vi "Remove XLSX last empty row.vi"(8 "Error In":errorcluster, 11 "Array in":string[][](array[string])) -> (0 "Error Out":errorcluster, 1 "Last Empty Row Removed":bool, 3 "Array out":string[][](array[string]))   [LabVIEW 2021, in "Files.lvlib"]
uses:
  <userlib>/_OpenG.lib/array/array.llb/Remove Duplicates from 1D Array (String)__ogtk.vi
  Files.lvlib
  <userlib>/_OpenG.lib/array/array.llb/openg_array.lvlib
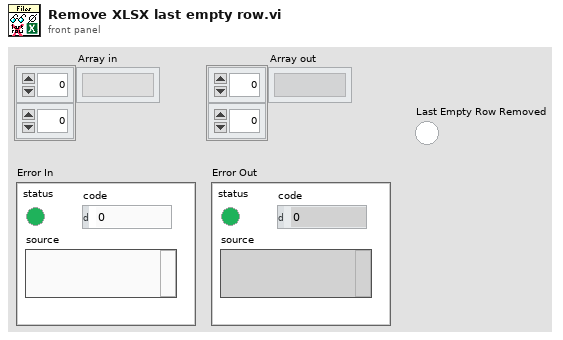
[diagram p1: front panel]
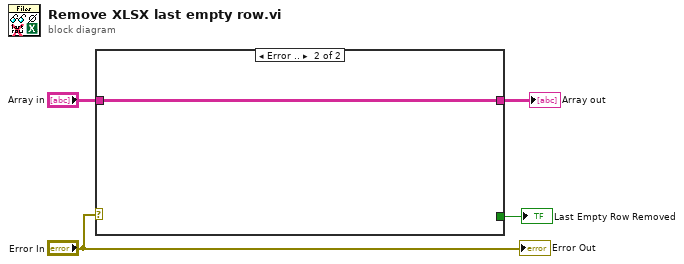
[diagram p0: block diagram]
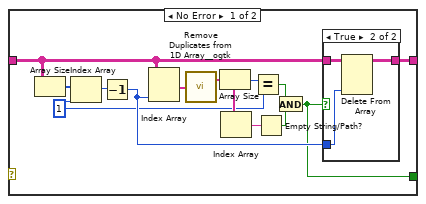
[diagram p2: hidden frame]
diagram:
  n1 = case shown="Error .." "Error In" {
    tunnel: "Array in" -> [w9 w22]
    tunnel: [w6 w22] -> w3
    tunnel: [w5 _] -> w2
    frame No Error {
      w12 = 1 ("index")
      n2 = Array Size(array=w9) -> (size(s)=w7:i32[])
      n3 = Index Array(array=w7, index=w12) -> (element=w8:i32)
      n4 = Decrement(x=w8) -> (x-1=w17:i32)
      n5 = Index Array(array=w9, index (col)=w17) -> (element=w10:string[])  [unwired: 1 in]
      n6 = call-poly <userlib>:"Remove Duplicates from 1D Array__ogtk.vi"("Input Array"=w10) -> ("Output Array"=w13:string[])  [unwired: 1 out]
      n7 = Array Size(array=w13) -> (size(s)=w11:i32)
      n8 = Index Array(array=w13) -> (element=w14:string)  [unwired: 1 in]
      n9 = Equal?(x=w11, y=w12) -> (x = y?=w15:bool)
      n10 = Empty String/Path?(string/path=w14) -> (empty?=w16:bool)
      n11 = And(x=w15, y=w16) -> (x .and. y?=w5:bool)
      n12 = case shown="True" w5 {
        tunnel: [w18 w21] -> w6
        tunnel: w9 -> [w18 w20]
        tunnel: w17 -> [_ w19]
        frame False {
        }
        frame True {
          n13 = Delete From Array(array=w20, index (col)=w19) -> (array with subset deleted=w21:string[][])  [unwired: 2 in, 1 out]
        }
      }
    }
    frame Error {
    }
  }
  "Array out" <- w3
  "Last Empty Row Removed" <- w2
  "Error Out" <- "Error In"
